vi "ds_error_handler.vi"(11 "Error Messaege":string) -> ()   [LabVIEW 2011]
uses:
  <vilib>/Rock Robotics/WPI/DriverStation/WPI_DriverStationStatusErrorCache.ctl
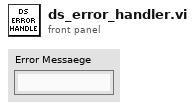
[diagram p1: front panel]
types:
  T1 = typedef "WPI_DriverStationStatusErrorCache.ctl" = enum16{"Get", "Set"}
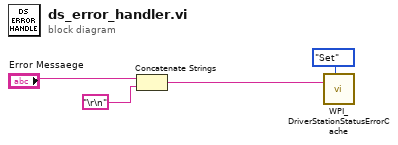
[diagram p0: block diagram]
diagram:
  n1 = Concatenate Strings("Error Messaege", "\r\n") -> (w1:string)
  n2 = call <vilib>:"WPI_DriverStationStatusErrorCache.vi"("StatusErrorCacheOp"=WPI_DriverStationStatusErrorCache."Set", "Error String"=w1) -> ()  [unwired: 10 out]
